vi "dfd_FXP Apply Gain.vi"(7 "FXPOPs":T1[](array[typedef]) {"source" items=["Coef a/k"=0, "Coef b/v"=7, "Input"=1, "Output"=2, "Multiplicand"=3, "Product"=4, "Sum"=5, "Delay"=6, "Gain"=8]}, 8 "filtering statistics in":T6(array[cluster]) {"statistics information"."min value" format="%.2f"; "statistics information"."max value" format="%.2f"; "Quantizer Source" items=["Coefficients a/k"=0, "Coefficients b/v"=7, "Input"=1, "Output"=2, "Multiplicand"=3, "Product"=4, "Sum"=5, "Delay"=6]}, 10 "gain":dbl, 11 "before-gain X":T3) -> (0 "filtering statistics out":T6(array[cluster]) {"statistics information"."min value" format="%.2f"; "statistics information"."max value" format="%.2f"; "Quantizer Source" items=["Coefficients a/k"=0, "Coefficients b/v"=7, "Input"=1, "Output"=2, "Multiplicand"=3, "Product"=4, "Sum"=5, "Delay"=6]}, 3 "after-gain X":T3)   [LabVIEW 2017, in "NI_DigFilter_FXP.lvlib"]
uses:
  <vilib>/addons/Digital Filter Design/NI_DigFilter_FXP.lvlib
  <vilib>/addons/Digital Filter Design/_Objects.llb/dfd_DFXP Data Type (vector).ctl
  <vilib>/addons/Digital Filter Design/_Objects.llb/DFD Quantization Sources.ctl
  <vilib>/addons/Digital Filter Design/_Objects.llb/DFD FXP Statistics Data.ctl
  <vilib>/addons/Digital Filter Design/_Objects.llb/dfd_DFXP Operation Parameter.ctl
  <vilib>/addons/Digital Filter Design/_Objects.llb/dfd_Internal Quantization Srcs.ctl
  <vilib>/addons/Digital Filter Design/NI_DigFilterLicensed.lvlib
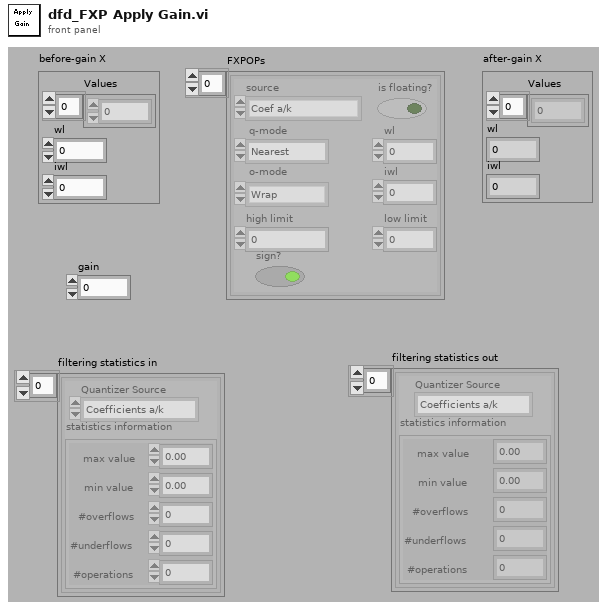
[diagram p1: front panel]
types:
  T1 = typedef "dfd_DFXP Operation Parameter.ctl" = cluster{"source":T2, "is floating?":bool, "o-mode":enum16{"Saturation", "Wrap"}, "q-mode":enum16{"Nearest", "Truncation"}, "wl":i16, "high limit":i64, "low limit":i64, "iwl":i16, "sign?":bool}
  T2 = typedef "NI_DigFilterLicensed.lvlib/dfd_Internal Quantization Srcs.ctl" = u16
  T3 = typedef "dfd_DFXP Data Type (vector).ctl" = cluster{"Values":i64[], "wl":i16, "iwl":i16}
  T4 = typedef "NI_DigFilterLicensed.lvlib/DFD Quantization Sources.ctl" = u16
  T5 = typedef "NI_DigFilterLicensed.lvlib/DFD FXP Statistics Data.ctl" = cluster{"max value":ext, "min value":ext, "#overflows":i32, "#underflows":i32, "#operations":i32}
  T6 = cluster{"Quantizer Source":T4, "statistics information":T5}[]
  T7 = typedef "dfd_DFXP Data Type (scaler).ctl" = cluster{"value":i64, "wl":i16, "iwl":i16, "Signed":bool}
  T8 = cluster{"Quantizer Source":T4, "statistics information":T5}
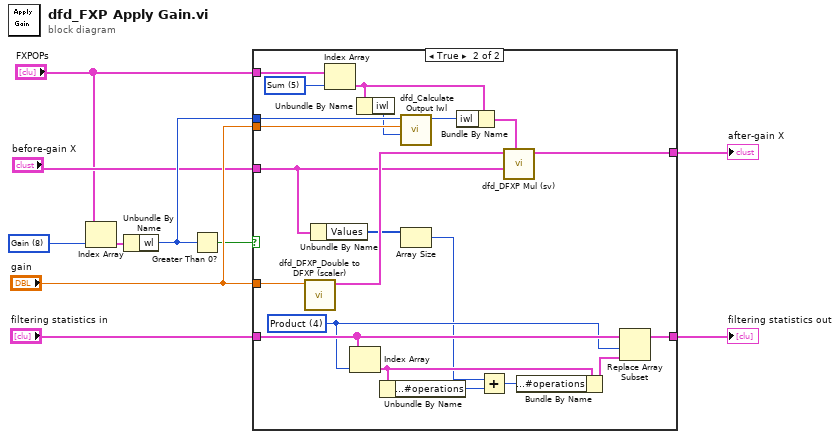
[diagram p0: block diagram]
diagram:
  w8 = T2 8 items=["Coef a/k"=0, "Coef b/v"=7, "Input"=1, "Output"=2, "Multiplicand"=3, "Product"=4, "Sum"=5, "Delay"=6, "Gain"=8] ("source")
  n1 = Index Array(array="FXPOPs", index=w8) -> (element=w5:T1)
  n2 = Unbundle By Name(w5) -> ("wl"=w7:i16)
  n3 = Greater Than 0?(x=w7) -> (x > 0?=w4:bool)
  n4 = case shown="True" w4 {
    tunnel: "before-gain X" -> [w12 w15]
    tunnel: [w12 w17] -> w2
    tunnel: "filtering statistics in" -> [w11 w33]
    tunnel: [w11 w32] -> w9
    tunnel: "gain" -> [_ w19]
    tunnel: "FXPOPs" -> [_ w26]
    tunnel: w7 -> [_ w24]
    tunnel: "gain" -> [_ w23]
    frame False {
    }
    frame True {
      w25 = T2 5 items=["Coef a/k"=0, "Coef b/v"=7, "Input"=1, "Output"=2, "Multiplicand"=3, "Product"=4, "Sum"=5, "Delay"=6, "Gain"=8] ("source")
      w31 = T2 4 items=["Coef a/k"=0, "Coef b/v"=7, "Input"=1, "Output"=2, "Multiplicand"=3, "Product"=4, "Sum"=5, "Delay"=6, "Gain"=8] ("source")
      n5 = call <vilib>:"dfd_DFXP_Double to DFXP (scaler).vi"("Double"=w19) -> ("FXP"=w16:T7)  [unwired: 10 out]
      n6 = Unbundle By Name(w15) -> ("Values"=w14:i64[])
      n7 = Index Array(array=w26, index=w25) -> (element=w20:T1)
      n8 = Index Array(array=w33, index=w31) -> (element=w27:T8)
      n9 = Unbundle By Name(w20) -> ("iwl"=w22:i16)
      n10 = Unbundle By Name(w27) -> ("statistics information.#operations"=w28:i32)
      n11 = call <vilib>:"dfd_Calculate Output Iwl.vi"("sum iwl"=w22, "gain value"=w23, "gain wl"=w24) -> ("output iwl"=w21:i16)  [unwired: 8 out]
      n12 = Array Size(array=w14) -> (size(s)=w13:i32)
      n13 = Bundle By Name(cluster=w20, "iwl"=w21) -> (w18:T1)
      n14 = Add(x=w13, y=w28) -> (x+y=w30:i32)
      n15 = call <vilib>:"dfd_DFXP Mul (sv).vi"("op params"=w18, "Value in 2"=w15, "Value in"=w16) -> ("Value out"=w17:T3)  [unwired: 3 in, 5 out]
      n16 = Bundle By Name(cluster=w27, "statistics information.#operations"=w30) -> (w29:T8)
      n17 = Replace Array Subset(array=w33, new element=w29, index=w31) -> (w32:T6)
    }
  }
  "after-gain X" <- w2
  "filtering statistics out" <- w9
